vi "Dashboard Main.vi"() -> ()   [LabVIEW 2017]
uses:
  <vilib>/Utility/miscctls.llb/LVRowAndColumnTypeDef.ctl
  <vilib>/Rock Robotics/Network Tables/NT Write Boolean.vi
  <vilib>/Rock Robotics/WPI/Dashboard/WPI_DashboardLogging Global.vi
panel:
  out "timer":sgl(slide) scale=0.0..100.0
  in  "Camera Name":string(combo)="No Camera Selection"
  in  "Camera Settings":T1={"Frame Rate"=30, "Compression"=30, "Size"=1, "DB Camera Config"=FALSE} {"Frame Rate" scale=1.0..30.0; "Compression" scale=100.0..-1.0; "Size" items=["640x480", "320x240", "160x120"]}
  in  "TCP":refnum<k5>
  out "Robot IP":string
  out "Image Message":string="Timeout in Camera Communications"
  in  "Dashboard Tab":T2(tab)
  out "Gyro":dbl(knob) scale=0.0..360.0
  in  "Auto Wait (s)":dbl
  in  "Reverse Climber":bool
  in  "Start Side":i32(listbox)
  in  "Autonomous":i32(listbox)
  out "NT Connection":bool
  out "Mode":T3(ring)=enum."Auto Disabled"
  out "Camera Info":cluster{"Mbps LED":bool, "Mbps":dbl, "fps":dbl} {"fps" format="%#.1g"; "Mbps" format="%#.1g"}
  in  "Rec Mode":enum32{"Stop", "Record", "Playback"}(radio)
  in  "driveRampUpD":dbl
  in  "driveRampUpS":dbl
  in  "driveS3":dbl
  in  "driveD3":dbl
  in  "driveS2":dbl
  in  "turnS2":dbl
  in  "driveD2":dbl
  in  "driveS1":dbl
  in  "turnD2":dbl
  in  "turnS1":dbl
  in  "afterDriveWait":dbl
  in  "outtakeSpeed":dbl
  in  "intakeSpeed":dbl
  in  "climbCurLim":dbl
  in  "rightPos_D":dbl
  in  "rightPos_I":dbl
  in  "rightPos_P":dbl
  in  "leftPos_D":dbl
  in  "leftPos_I":dbl
  in  "leftPos_P":dbl
  in  "turn_D":dbl
  in  "turn_I":dbl
  in  "turn_P":dbl
  in  "rightDrive_F":dbl
  in  "leftDrive_F":dbl
  in  "rightDrive_D":dbl
  in  "rightDrive_I":dbl
  in  "rightDrive_P":dbl
  in  "leftDrive_D":dbl
  in  "leftDrive_I":dbl
  in  "leftDrive_P":dbl
  in  "configFile":path=path "C:/Users/lavre/Desktop/Robotics/Programming/2018 Programming/2018-Dashboard/docs/config_sample.json"
  in  "DB Camera Config":bool
  in  "Camera Settings Right":T4={"Frame Rate"=30, "Compression"=30, "Size"=1} {"Frame Rate" scale=1.0..30.0; "Compression" scale=100.0..-1.0; "Size" items=["640x480", "320x240", "160x120"]}
  in  "Camera Name Right":string(combo)="No Camera Selection"
  in  "Test Slider":dbl(slide) scale=0.0..100.0 scale format="%#_3g"
  in  "On/Off":bool caption="Solenoid"
  in  "Test Name":u16(ring) items=["Select the test to run..."]
  in  "Test Tree":string(tree)
  in  "Motor":cluster{"Value":dbl, "Enable":bool} {"Value" scale=-1.0..1.0 scale format="%#_3g"}
  out "Progress":T5 {"Test Progress" scale=0.0..100.0}
  in  "Rev/Fwd":cluster{"Forward":bool, "Reverse":bool}
  in  "Test Ring":u16(ring) items=["Monochrome", "Color"]
  out "Cmd Status":string
  in  "Execute Command":bool
  in  "Command Params":string[][](table)
  in  "Command Selection":i32(listbox)
  out "Tree":string(tree)
  out "Camera Image":T6(plugin-control)
  # "HW"
  # "Asterisks (*) mean that that auto is untested\nand should not be run in a competition setting"
  # "Velocity PID Constants"
  # "Auto Turn PID Constants"
  # "Auto Drive PID Constants"
  # "Auto Drive Ramp Constants"
  # "Tele-Op Constants"
  # "Auto Turn Ramp Constants"
  # "inches"
  # "Amps"
  # "inches"
  # "inches"
  # "S1: max speed (native units [1-4200])\nS2: bot speed (native units [1-4200])\nD2: angle from target at which to switch to S2 (in)"
  # "ms"
  # "HW"
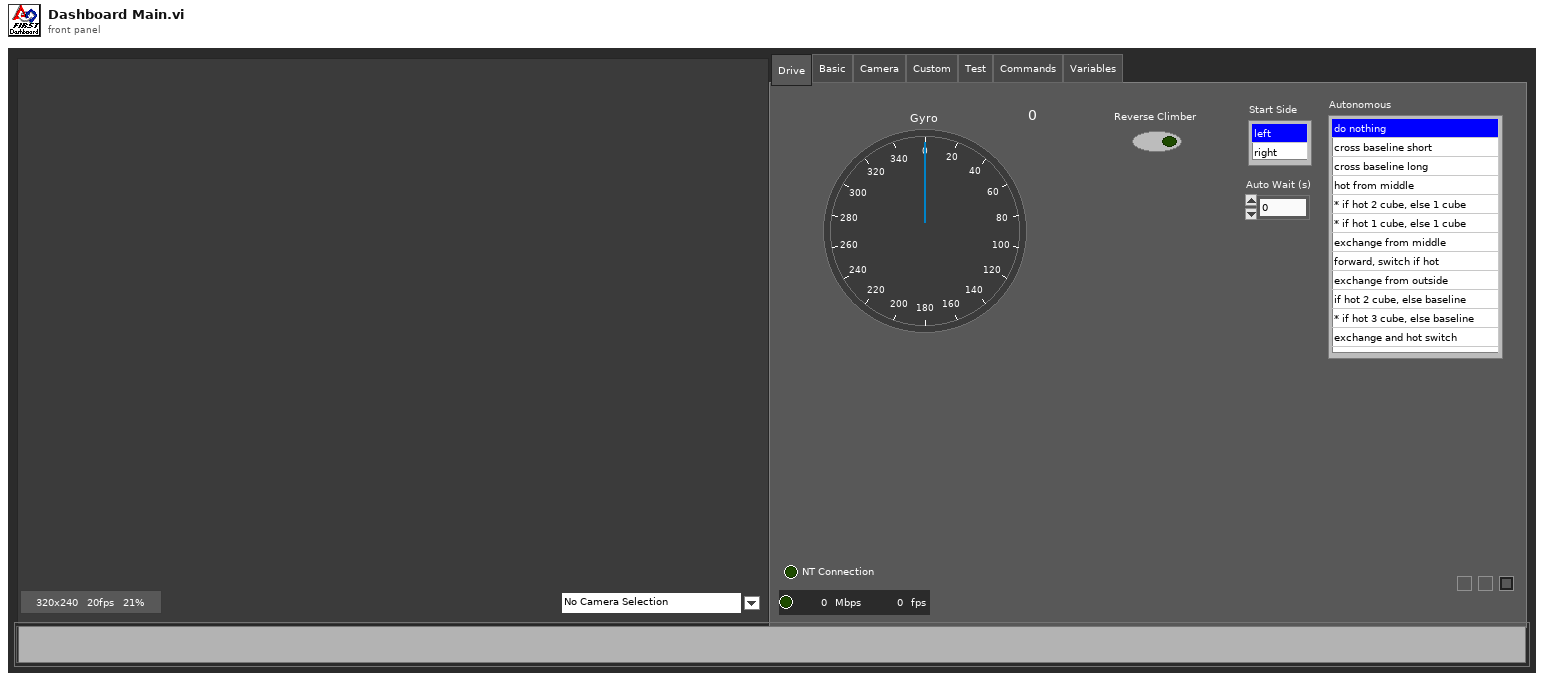
[diagram p1: front panel]
types:
  T1 = cluster{"Frame Rate":i32, "Compression":i32, "Size":u16, "DB Camera Config":bool}
  T2 = enum32{"Drive", "Basic", "Camera", "Custom", "Test", "Commands", "Variables"}
  T3 = enum8{"Tele-Op Disabled", "Tele-Op Enabled", "Auto Disabled", "Auto Enabled", "Test Disabled", "Test Enabled", "Disconnected", "No Code", "E-Stop"}
  T4 = cluster{"Frame Rate":i32, "Compression":i32, "Size":u16}
  T5 = cluster{"Test Progress":u8, "Test Progress Text":string}
  T6 = typedef "IMAQ Image.ctl" = refnum<image>
  T7 = cluster{"Save Path":path, "Interval (s)":dbl, "Keep":i32}
  T8 = enum32{"Drive", "Camera", "Basic", "Custom", "Test", "Commands", "Checklist", "Variables"}
  T9 = typedef "Image Type" = u32
  T10 = cluster{"IDs":cluster{"RPC field ID":u16, "Unique ID":u16}, "String":string}
  T11 = cluster{"velocityPIDConsts":cluster{"leftDrive_P":dbl, "leftDrive_I":dbl, "leftDrive_D":dbl, "leftDrive_F":dbl, "rightDrive_P":dbl, "rightDrive_I":dbl, "rightDrive_D":dbl, "rightDrive_F":dbl}, "teleOpConsts":cluster{"climbCurLim":dbl, "intakeSpeed":dbl, "outtakeSpeed":dbl, "reverseClimber":bool}, "autoTurnPIDConsts":cluster{"turn_P":dbl, "turn_I":dbl, "turn_D":dbl}, "autoTurnRampConsts":cluster{"turnS1":dbl, "turnD2":dbl, "turnS2":dbl}, "autoDrivePIDConsts":cluster{"leftPos_P":dbl, "leftPos_I":dbl, "leftPos_D":dbl, "rightPos_P":dbl, "rightPos_I":dbl, "rightPos_D":dbl}, "autoDriveRampConsts":cluster{"driveS1":dbl, "driveD2":dbl, "driveS2":dbl, "driveD3":dbl, "driveS3":dbl, "autoDriveRampUpS":dbl, "autoDriveRampUpD":dbl, "afterDriveWait":dbl}}
  T12 = cluster{"leftDrive_P":dbl, "leftDrive_I":dbl, "leftDrive_D":dbl, "leftDrive_F":dbl, "rightDrive_P":dbl, "rightDrive_I":dbl, "rightDrive_D":dbl, "rightDrive_F":dbl}
  T13 = cluster{"climbCurLim":dbl, "intakeSpeed":dbl, "outtakeSpeed":dbl, "reverseClimber":bool}
  T14 = cluster{"turn_P":dbl, "turn_I":dbl, "turn_D":dbl}
  T15 = cluster{"turnS1":dbl, "turnD2":dbl, "turnS2":dbl}
  T16 = cluster{"leftPos_P":dbl, "leftPos_I":dbl, "leftPos_D":dbl, "rightPos_P":dbl, "rightPos_I":dbl, "rightPos_D":dbl}
  T17 = cluster{"driveS1":dbl, "driveD2":dbl, "driveS2":dbl, "driveD3":dbl, "driveS3":dbl, "autoDriveRampUpS":dbl, "autoDriveRampUpD":dbl, "afterDriveWait":dbl}
  T18 = cluster{"Error Strings":string, "Disable Counts":cluster{u16, u16}, "Rail Faults":cluster{u16, u16, u16}, "Robot IP":string, "DB Mode":u8, "Event Info":cluster{"Name":string, "Type":u8, "Number":u16, "Replay":u8}}
  T19 = cluster{"Storage":cluster{"Disk Free":u64, "RAM Block":u32, "RAM free":u32}, "CPU Utilization":cluster{"CPU % ISR":sgl, "CPU % Time Crit":sgl, "CPU % Timed Str":sgl, "CPU % High":sgl, "CPU % Above":sgl, "CPU % Normal":sgl, "CPU % Low":sgl}, "CAN":cluster{"% Bus Utilization":sgl, "Bus Off Cnt":u32, "TX_FIFO Full Cnt":u32, "Receive Error Cnt":u8, "Transmit Error Cnt":u8}, "HID":cluster{"HID Outputs":u32, "Rumble Low":u16, "Rumble High":u16}[]}
  T20 = cluster{"Status bits":cluster{"Test Mode":bool, "Autonomous":bool, "Enabled":bool, "Code Start":bool, "Brownout":bool, "Reserved 2":bool, "Reserved 3":bool, "E-Stop":bool}, "Code Trace":cluster{"Disabled":bool, "TeleOp":bool, "Auto":bool, "Test":bool}, "Controller Type":enum16{"unknown", "cRIO", "roboRio"}, "Code?":enum16{"unknown", "noCode", "code"}, "Battery V":dbl}
  T21 = cluster{"Control Bits":cluster{"TestMode":bool, "Autonomous":bool, "Enabled":bool, "FMS Present":bool, bool, bool, bool, "E-Stop":bool}, "Team Station ":u8, "Countdown":sgl, "Joystick Values":cluster{"Axes":dbl[], "Buttons":bool[], "POVs":i16[]}[]}
  T22 = cluster{"Camera Name":string, string, "Saved DB Images Info":cluster{"Save Path":path, "Interval (s)":dbl, "Keep":i32}}
  T23 = cluster{"Camera Name Right":string, string, "Saved DB Images Info":cluster{"Save Path":path, "Interval (s)":dbl, "Keep":i32}}
  T24 = cluster{"Operation":enum16{"Update", "Clear"}, "Color Box":u32}[]
  T25 = cluster{"Image Size":bool, "Image Type":bool, "Pixel Value":bool, "ROI Information":bool, "Zoom Factor":bool}
  T26 = cluster{"Operation":enum16{"Update", "Clear"}, "Color Box":u32}
  T27 = typedef "LVRowAndColumnTypeDef.ctl" = cluster{"Row":i32, "Column":i32}
  T28 = cluster{"Shift":bool, "Ctrl":bool, "Alt":bool, "Cmd":bool, "Opt":bool}
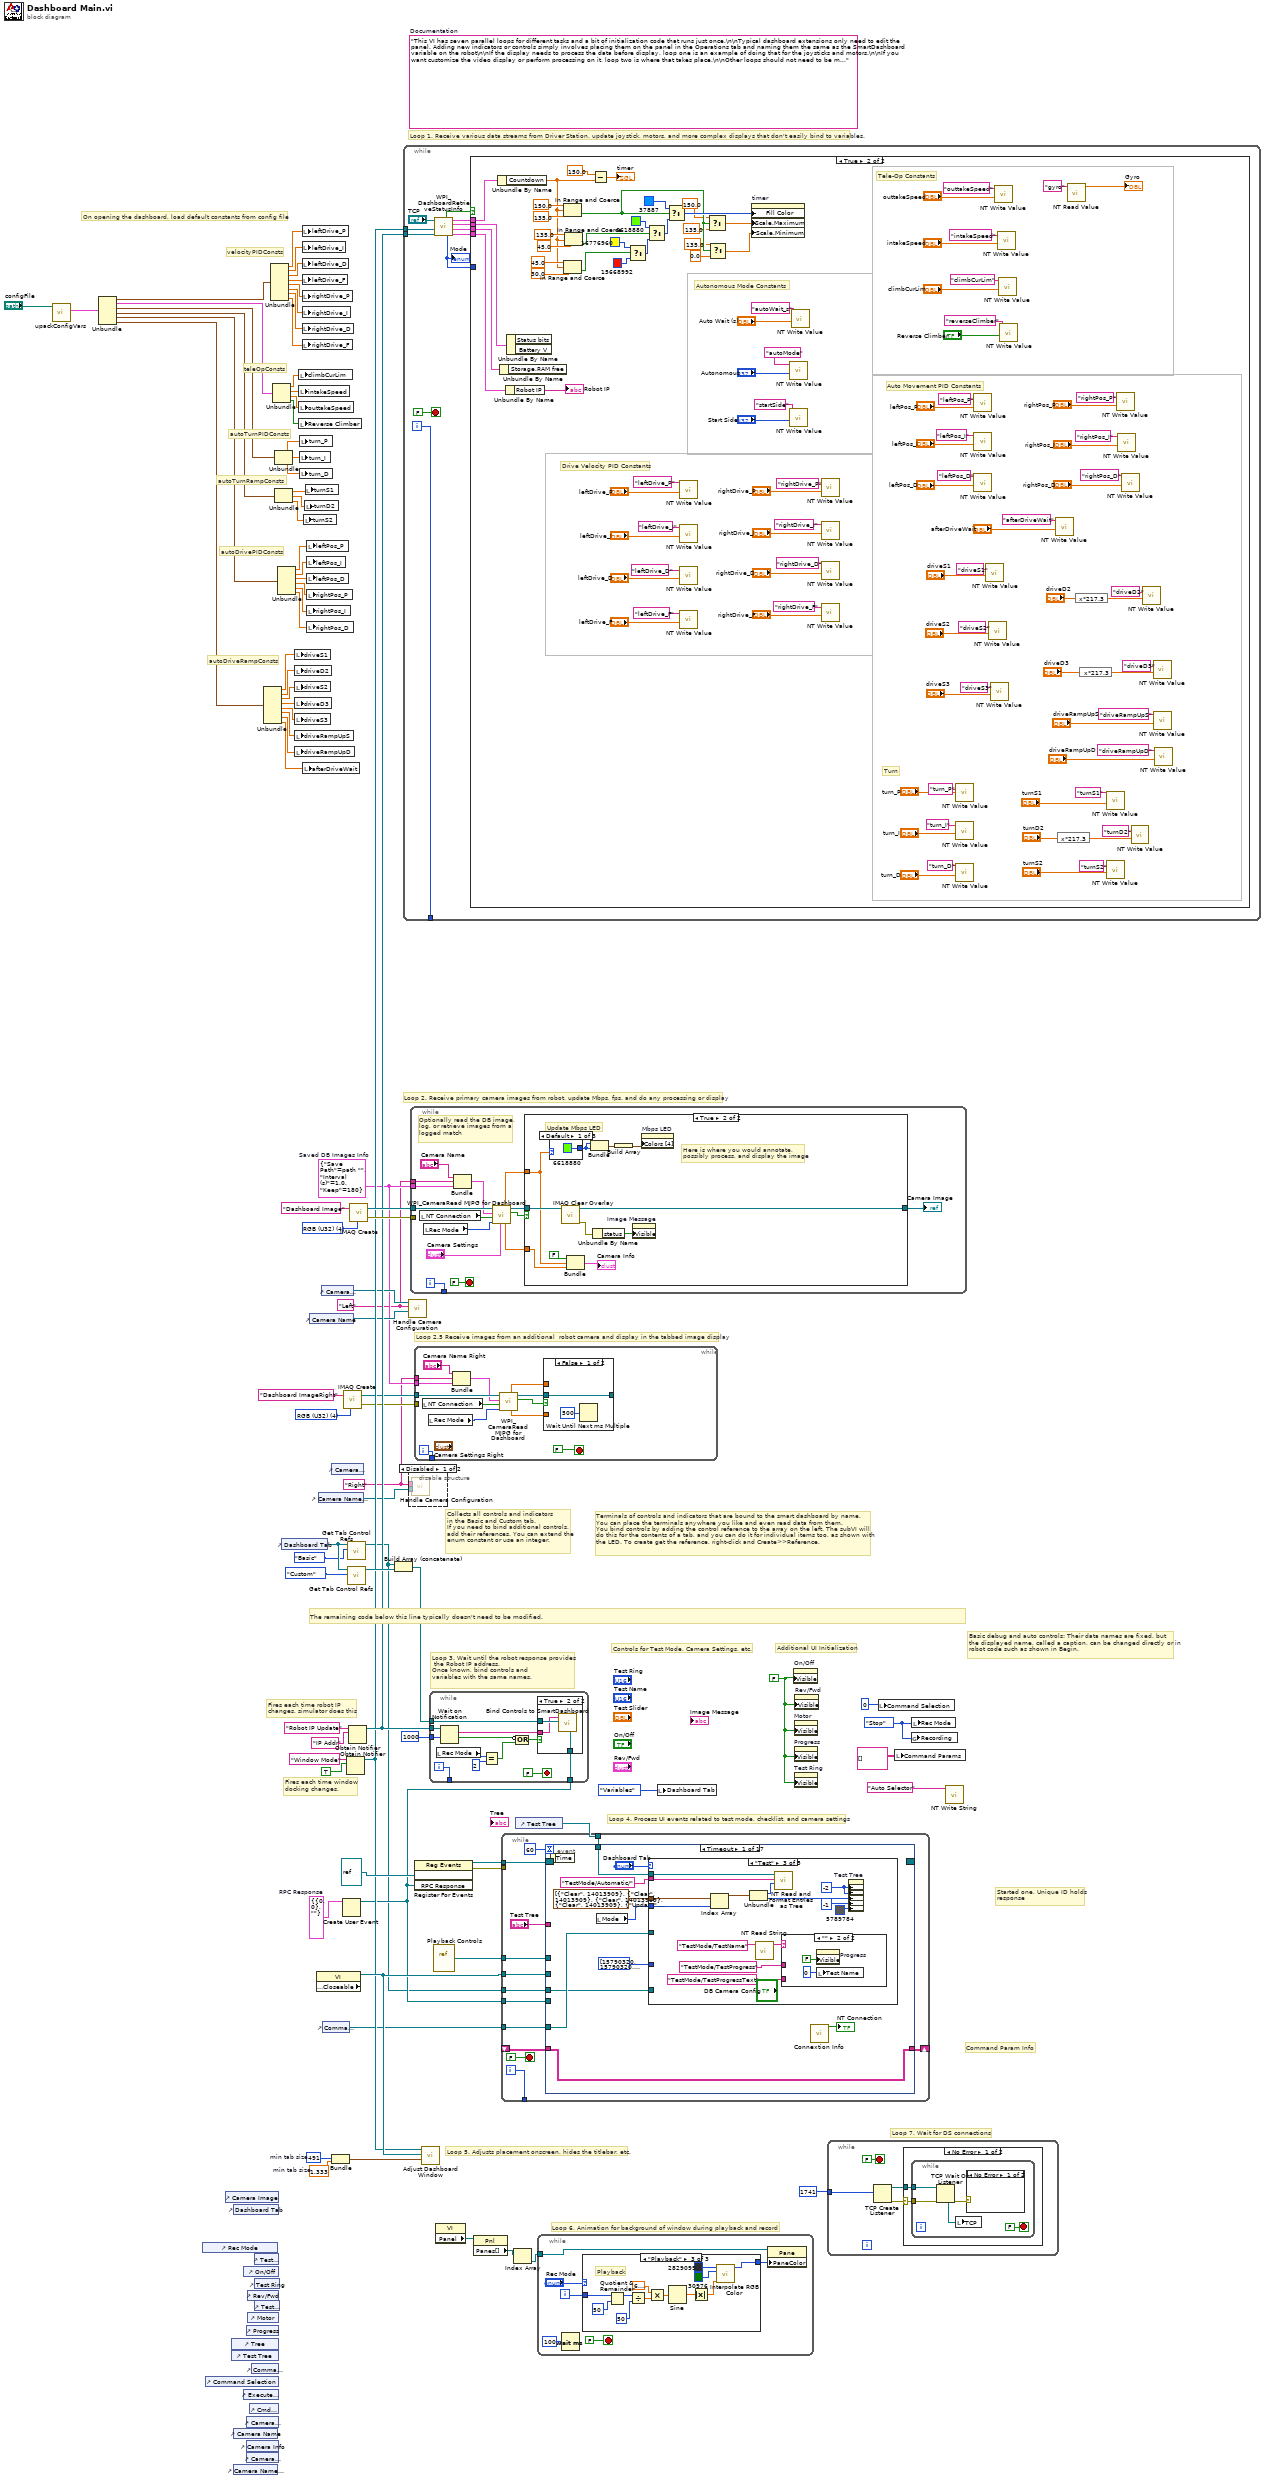
[diagram p0: block diagram]
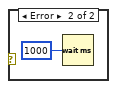
[diagram p4: hidden frame]
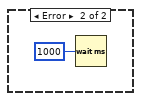
[diagram p5: hidden frame]
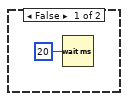
[diagram p6: hidden frame]
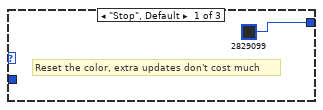
[diagram p7: hidden frame]
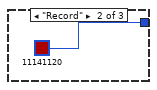
[diagram p8: hidden frame]
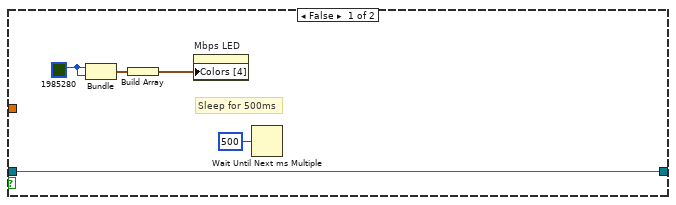
[diagram p10: hidden frame]
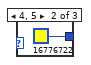
[diagram p11: hidden frame]
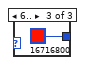
[diagram p12: hidden frame]
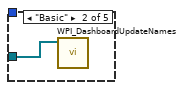
[diagram p14: hidden frame]
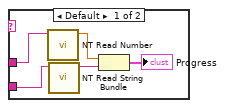
[diagram p15: hidden frame]
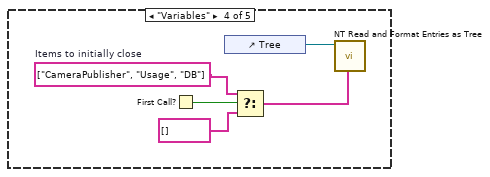
[diagram p16: hidden frame]
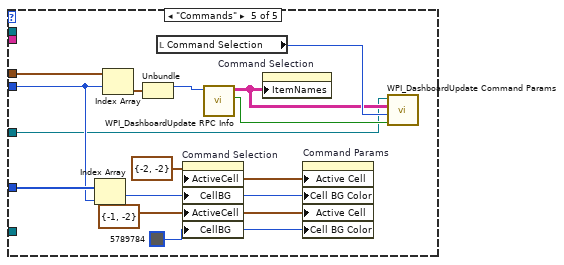
[diagram p17: hidden frame]
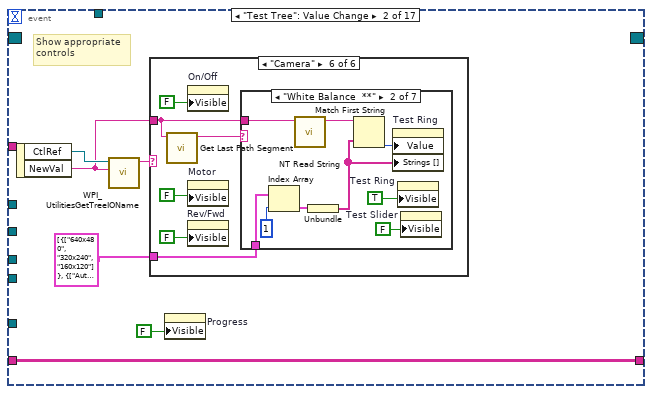
[diagram p18: hidden frame]
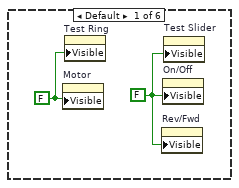
[diagram p19: hidden frame]
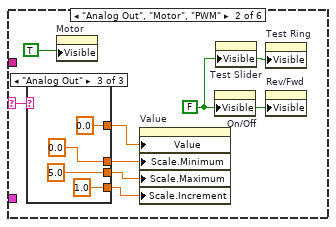
[diagram p20: hidden frame]
diagram:
  w43 = T7 {"Save Path"=path "", "Interval (s)"=1.0, "Keep"=180}  # Saved DB Images Info
  w42 = "Right"
  w41 = "Left"
  w49 = T9 4 items=["Grayscale (U8)", "Grayscale (I16)", "Grayscale (SGL)", "Complex (CSG)", "RGB (U32)", "HSL (U32)", "RGB (U64)"] ("Image Type")
  w59 = T10 {"IDs"={"RPC field ID"=0, "Unique ID"=0}, "String"=""}  # RPC Response
  w67 = 491  # min tab size
  w66 = 1.333  # min tab size
  w72 = enum32{"Stop", "Record", "Playback"}."Stop" ("Rec Mode")
  w64 = FALSE ("Visible")
  (unwired) "This VI has seven parallel loops for different tasks and a bit of initialization code that runs just once.\n\nTypical dashboard extensions only need to edit the panel. Adding new indicators or controls simply involves placing them on the panel in the Operations tab and naming them the same as the SmartDashboard variable on the robot\n\nIf the display needs to process the data before display, loop one is an example of doing that for the joysticks and motors.\n\nIf you want customize the video display or perform processing on it, loop two is where that takes place.\n\nOther loops should not need to be modified. They are pretty standard, and document the task they perform."  # Documentation
  w89 = T9 4 items=["Grayscale (U8)", "Grayscale (I16)", "Grayscale (SGL)", "Complex (CSG)", "RGB (U32)", "HSL (U32)", "RGB (U64)"] ("Image Type")
  # "autoDriveRampConsts"
  # "autoDrivePIDConsts"
  # "autoTurnRampConsts"
  # "autoTurnPIDConsts"
  # "teleOpConsts"
  # "velocityPIDConsts"
  # "On opening the dashboard, load default constants from config file"
  # "Collects all controls and indicators\nin the Basic and Custom tab.\nIf you need to bind additional controls,\nadd their references. You can extend the\nenum constant or use an integer."
  # "Loop 2.5 Receive images from an additional  robot camera and display in the tabbed image display"
  # "Command Param Info"
  # "Started one, Unique ID holds\nresponse"
  # "Loop 7. Wait for DS connections"
  # "Basic debug and auto controls: Their data names are fixed, but\nthe displayed name, called a caption, can be changed directly or in\nrobot code such as shown in Begin."
  # "Controls for Test Mode, Camera Settings, etc."
  # "Additional UI Initialization"
  # "Loop 6. Animation for background of window during playback and record"
  # "Fires each time robot IP\nchanges, simulator does this"
  # "Fires each time window\ndocking changes."
  # "The remaining code below this line typically doesn't need to be modified."
  # "Loop 4. Process UI events related to test mode, checklist, and camera settings"
  # "Terminals of controls and indicators that are bound to the smart dashboard by name.\nYou can place the terminals anywhere you like and even read data from them.\nYou bind controls by adding the control reference to the array on the left. The subVI will\ndo this for the contents of a tab, and you can do it for individual items too, as shown with\nthe LED. To create get the reference, right-click and Create>>Reference."
  # "Loop 3. Wait until the robot response provides\n the Robot IP address.\nOnce known, bind controls and\nvariables with the same names."
  # "Loop 5. Adjusts placement onscreen, hides the titlebar, etc."
  # "Loop 1. Receive various data streams from Driver Station, update joystick, motors, and more complex displays that don't easily bind to variables."
  # "Loop 2. Receive primary camera images from robot, update Mbps, fps, and do any processing or display"
  n1 = call "upackConfigVars.vi"("file"="configFile") -> ("configVars"=w1:T11)  [unwired: 10 in]
  n2 = Unbundle(w1) -> ("velocityPIDConsts"=w31:T12, "teleOpConsts"=w30:T13, "autoTurnPIDConsts"=w25:T14, "autoTurnRampConsts"=w21:T15, "autoDrivePIDConsts"=w17:T16, "autoDriveRampConsts"=w16:T17)
  n3 = control-ref of="Rec Mode"() -> ()  [unwired: 1 out]
  n4 = control-ref of="Command Selection"() -> ()  [unwired: 1 out]
  n5 = control-ref of="Camera Image"() -> ()  [unwired: 1 out]
  n6 = control-ref of="Tree"() -> ()  [unwired: 1 out]
  n7 = control-ref of="Test Tree"() -> ()  [unwired: 1 out]
  n8 = control-ref of="Dashboard Tab"() -> ()  [unwired: 1 out]
  n9 = control-ref of="Camera Name"() -> ()  [unwired: 1 out]
  n10 = control-ref of="Camera Name Right"() -> ()  [unwired: 1 out]
  n11 = control-ref of="Execute Command"() -> ()  [unwired: 1 out]
  n12 = control-ref of="On/Off"() -> ()  [unwired: 1 out]
  n13 = control-ref of="Progress"() -> ()  [unwired: 1 out]
  n14 = control-ref of="Camera Settings"() -> ()  [unwired: 1 out]
  n15 = control-ref of="Camera Info"() -> ()  [unwired: 1 out]
  n16 = control-ref of="Camera Settings Right"() -> ()  [unwired: 1 out]
  n17 = control-ref of="Rev/Fwd"() -> ()  [unwired: 1 out]
  n18 = control-ref of="Motor"() -> ()  [unwired: 1 out]
  n19 = control-ref of="Cmd Status"() -> ()  [unwired: 1 out]
  n20 = control-ref of="Command Params"() -> ()  [unwired: 1 out]
  n21 = control-ref of="Test Slider"() -> ()  [unwired: 1 out]
  n22 = control-ref of="Test Ring"() -> ()  [unwired: 1 out]
  n23 = control-ref of="Test Name"() -> ()  [unwired: 1 out]
  n24 = Unbundle(w16) -> ("driveS1"=w2:dbl, "driveD2"=w3:dbl, "driveS2"=w4:dbl, "driveD3"=w5:dbl, "driveS3"=w6:dbl, "autoDriveRampUpS"=w7:dbl, "autoDriveRampUpD"=w8:dbl, "afterDriveWait"=w9:dbl)
  n25 = Unbundle(w31) -> ("leftDrive_P"=w39:dbl, "leftDrive_I"=w38:dbl, "leftDrive_D"=w37:dbl, "leftDrive_F"=w36:dbl, "rightDrive_P"=w35:dbl, "rightDrive_I"=w34:dbl, "rightDrive_D"=w33:dbl, "rightDrive_F"=w32:dbl)
  n26 = Unbundle(w30) -> ("climbCurLim"=w29:dbl, "intakeSpeed"=w28:dbl, "outtakeSpeed"=w27:dbl, "reverseClimber"=w26:bool)
  n27 = Unbundle(w25) -> ("turn_P"=w24:dbl, "turn_I"=w23:dbl, "turn_D"=w22:dbl)
  n28 = Unbundle(w21) -> ("turnS1"=w20:dbl, "turnD2"=w18:dbl, "turnS2"=w19:dbl)
  n29 = Unbundle(w17) -> ("leftPos_P"=w15:dbl, "leftPos_I"=w14:dbl, "leftPos_D"=w12:dbl, "rightPos_P"=w13:dbl, "rightPos_I"=w11:dbl, "rightPos_D"=w10:dbl)
  n30 = control-ref of="Dashboard Tab"() -> (w70:refnum<vi>)
  n31 = local write "driveS1"(w2) -> ()
  n32 = local write "driveD2"(w3) -> ()
  n33 = local write "driveS2"(w4) -> ()
  n34 = local write "driveD3"(w5) -> ()
  n35 = local write "driveS3"(w6) -> ()
  n36 = local write "driveRampUpS"(w7) -> ()
  n37 = local write "driveRampUpD"(w8) -> ()
  n38 = local write "climbCurLim"(w29) -> ()
  n39 = local write "intakeSpeed"(w28) -> ()
  n40 = local write "outtakeSpeed"(w27) -> ()
  n41 = local write "Reverse Climber"(w26) -> ()
  n42 = local write "turn_P"(w24) -> ()
  n43 = local write "turn_I"(w23) -> ()
  n44 = local write "turn_D"(w22) -> ()
  n45 = local write "leftDrive_P"(w39) -> ()
  n46 = local write "leftDrive_I"(w38) -> ()
  n47 = local write "leftDrive_D"(w37) -> ()
  n48 = local write "leftDrive_F"(w36) -> ()
  n49 = local write "rightDrive_P"(w35) -> ()
  n50 = local write "rightDrive_I"(w34) -> ()
  n51 = local write "rightDrive_D"(w33) -> ()
  n52 = local write "rightDrive_F"(w32) -> ()
  n53 = local write "afterDriveWait"(w9) -> ()
  n54 = local write "turnS2"(w19) -> ()
  n55 = local write "turnD2"(w18) -> ()
  n56 = local write "turnS1"(w20) -> ()
  n57 = local write "leftPos_P"(w15) -> ()
  n58 = local write "leftPos_I"(w14) -> ()
  n59 = local write "leftPos_D"(w12) -> ()
  n60 = local write "rightPos_P"(w13) -> ()
  n61 = local write "rightPos_I"(w11) -> ()
  n62 = local write "rightPos_D"(w10) -> ()
  n63 = control-ref of="Camera Name"() -> (w53:refnum<vi>)
  n64 = property class="VI" props=["Front Panel.Closeable"]() -> (reference out=w71:refnum<vi>)  [unwired: 2 in, 2 out]
  n65 = control-ref of="Camera Name Right"() -> (w46:refnum<vi>)
  n66 = control-ref of="Camera Settings"() -> (w54:refnum<vi>)
  n67 = control-ref of="Command Params"() -> (w55:refnum<vi>)
  n68 = control-ref of="Camera Settings Right"() -> ()  [unwired: 1 out]
  n69 = Bundle("min tab size"=w67, "min tab size"=w66) -> (w65:cluster{"min tab size":i32, "min tab size":dbl})  [unwired: 1 in]
  n70 = Create User Event(user event datatype=w59) -> (user event=w56:refnum<user-event>)  [unwired: 1 in, 1 out]
  n71 = call "IMAQ Create"("Image Name"="Dashboard ImageRight", "Image Type"=w49) -> ("New Image"=w48:T6, "error out"=w47:errorcluster)  [unwired: 2 in, 1 out]
  n72 = Obtain Notifier(name (unnamed)="Window Mode", notification data type=TRUE) -> (notifier out=w62:refnum<notifier>)  [unwired: 2 in, 2 out]
  n73 = call <vilib>:"Get Tab Control Refs.vi"("Page Index"=T8."Basic" ("Dashboard Tab"), "TabControl in"=w70) -> ("ControlsOnPage"=w52:refnum<vi>[])  [unwired: 9 in]
  n74 = call <vilib>:"Get Tab Control Refs.vi"("Page Index"=T8."Custom" ("Dashboard Tab"), "TabControl in"=w70) -> ("ControlsOnPage"=w69:refnum<vi>[])  [unwired: 9 in]
  n75 = Obtain Notifier(name (unnamed)="Robot IP Update", notification data type="IP Addr" ("name (unnamed)")) -> (notifier out=w63:refnum<notifier>)  [unwired: 2 in, 2 out]
  n76 = call "IMAQ Create"("Image Name"="Dashboard Image", "Image Type"=w89) -> ("New Image"=w87:T6, "error out"=w86:errorcluster)  [unwired: 2 in, 1 out]
  n77 = Build Array (concatenate)(w52, w69) -> (w68:refnum<vi>[])
  n78 = while {
    tunnel: [w99] -> _
    tunnel: w63 -> [w93]
    tunnel: w62 -> [w90]
    i -> [w99]
    stop <- FALSE stop-if-true
    n79 = call <vilib>:"WPI_DashboardRetrieveStatusInfo.vi"("Binding Refnum"=w93, "Window Mode Notifier"=w90, "TCP Cnx"="TCP") -> ("Power and Errors"=w94:T18, "Robot Metrics"=w97:T19, "Status Info"=w98:T20, "Control Info"=w95:T21, "Robot Mode"=w92:T3, "Process?"=w96:bool)  [unwired: 3 in]
    "Mode" <- w92
    n80 = case shown="True" w96 {
      tunnel: w98 -> [_ w206]
      tunnel: w97 -> [_ w205]
      tunnel: w95 -> [_ w204]
      tunnel: w94 -> [_ w203]
      tunnel: w92 -> [_ _]
      frame False {
        n81 = Wait (ms)(milliseconds to wait=u32 20) -> ()  [unwired: 1 out]
      }
      frame True {
        # "Turn"
        # "Auto Movement PID Constants"
        # "Drive Velocity PID Constants"
        # "Autonomous Mode Constants"
        # "Tele-Op Constants"
        n82 = Unbundle By Name(w204) -> ("Countdown"=w178:sgl)
        n83 = Unbundle By Name(w205) -> ()  [unwired: 1 out]
        n84 = Unbundle By Name(w203) -> ("Robot IP"=→"Robot IP":string)
        n85 = Unbundle By Name(w206) -> ()  [unwired: 2 out]
        n86 = In Range and Coerce(upper limit=150.0, x=w178, lower limit=135.0) -> (In Range?=w184:bool)  [unwired: 1 out]
        n87 = In Range and Coerce(upper limit=45.0, x=w178, lower limit=30.0) -> (In Range?=w189:bool)  [unwired: 1 out]
        n88 = In Range and Coerce(upper limit=135.0, x=w178, lower limit=45.0) -> (In Range?=w188:bool)  [unwired: 1 out]
        n89 = Subtract(x=sgl 150.0, y=w178) -> (x-y=→"timer":sgl)
        n90 = Select(t=u32 16776960 ("Color Box"), s=w189, f=u32 15668992 ("Color Box")) -> (s? t:f=w196:u32)
        n91 = Select(t=u32 6618880 ("Color Box"), s=w188, f=w196) -> (s? t:f=w198:u32)
        n92 = Select(t=u32 37887 ("Color Box"), s=w184, f=w198) -> (s? t:f=w187:u32)
        n93 = call-poly <vilib>:"NT Write Value.vi"("Numeric"="leftDrive_P", "Name"="leftDrive_P") -> ()  [unwired: 9 in, 1 out]
        n94 = call-poly <vilib>:"NT Write Value.vi"("Numeric"="leftDrive_I", "Name"="leftDrive_I") -> ()  [unwired: 9 in, 1 out]
        n95 = call-poly <vilib>:"NT Write Value.vi"("Numeric"="leftDrive_D", "Name"="leftDrive_D") -> ()  [unwired: 9 in, 1 out]
        n96 = call-poly <vilib>:"NT Write Value.vi"("Numeric"="leftDrive_F", "Name"="leftDrive_F") -> ()  [unwired: 9 in, 1 out]
        n97 = Select(t=150.0, s=w184, f=135.0) -> (s? t:f=w186:dbl)
        n98 = Select(t=135.0, s=w184, f=0.0) -> (s? t:f=w185:dbl)
        n99 = property on="timer" class="Slide (strict)"("Fill Color"=w187, "Scale.Maximum"=w186, "Scale.Minimum"=w185) -> ()  [unwired: 2 in, 2 out]
        n100 = call-poly <vilib>:"NT Write Value.vi"("Numeric"="Autonomous", "Name"="autoMode") -> ()  [unwired: 9 in, 1 out]
        n101 = call-poly <vilib>:"NT Write Value.vi"("Numeric"="Start Side", "Name"="startSide") -> ()  [unwired: 9 in, 1 out]
        n102 = call-poly <vilib>:"NT Write Value.vi"("Numeric"="Auto Wait (s)", "Name"="autoWait_s") -> ()  [unwired: 9 in, 1 out]
        n103 = call-poly <vilib>:"NT Write Value.vi"("Numeric"="rightDrive_P", "Name"="rightDrive_P") -> ()  [unwired: 9 in, 1 out]
        n104 = call-poly <vilib>:"NT Write Value.vi"("Numeric"="rightDrive_I", "Name"="rightDrive_I") -> ()  [unwired: 9 in, 1 out]
        n105 = call-poly <vilib>:"NT Write Value.vi"("Numeric"="rightDrive_D", "Name"="rightDrive_D") -> ()  [unwired: 9 in, 1 out]
        n106 = call-poly <vilib>:"NT Write Value.vi"("Numeric"="rightDrive_F", "Name"="rightDrive_F") -> ()  [unwired: 9 in, 1 out]
        n107 = call-poly <vilib>:"NT Write Value.vi"("Numeric"="turn_P", "Name"="turn_P") -> ()  [unwired: 9 in, 1 out]
        n108 = call-poly <vilib>:"NT Write Value.vi"("Numeric"="turn_I", "Name"="turn_I") -> ()  [unwired: 9 in, 1 out]
        n109 = call-poly <vilib>:"NT Write Value.vi"("Numeric"="turn_D", "Name"="turn_D") -> ()  [unwired: 9 in, 1 out]
        n110 = call-poly <vilib>:"NT Write Value.vi"("Numeric"="leftPos_P", "Name"="leftPos_P") -> ()  [unwired: 9 in, 1 out]
        n111 = call-poly <vilib>:"NT Write Value.vi"("Numeric"="leftPos_I", "Name"="leftPos_I") -> ()  [unwired: 9 in, 1 out]
        n112 = call-poly <vilib>:"NT Write Value.vi"("Numeric"="leftPos_D", "Name"="leftPos_D") -> ()  [unwired: 9 in, 1 out]
        n113 = call-poly <vilib>:"NT Write Value.vi"("Numeric"="driveS1", "Name"="driveS1") -> ()  [unwired: 9 in, 1 out]
        n114 = call-poly <vilib>:"NT Write Value.vi"("Numeric"="driveS2", "Name"="driveS2") -> ()  [unwired: 9 in, 1 out]
        n115 = call-poly <vilib>:"NT Write Value.vi"("Numeric"="driveS3", "Name"="driveS3") -> ()  [unwired: 9 in, 1 out]
        n116 = call-poly <vilib>:"NT Write Value.vi"("Numeric"="outtakeSpeed", "Name"="outtakeSpeed") -> ()  [unwired: 9 in, 1 out]
        n117 = call-poly <vilib>:"NT Write Value.vi"("Numeric"="intakeSpeed", "Name"="intakeSpeed") -> ()  [unwired: 9 in, 1 out]
        n118 = call-poly <vilib>:"NT Write Value.vi"("Numeric"="climbCurLim", "Name"="climbCurLim") -> ()  [unwired: 9 in, 1 out]
        n119 = call-poly <vilib>:"NT Write Value.vi"("Boolean"="Reverse Climber", "Name"="reverseClimber") -> ()  [unwired: 9 in, 1 out]
        n120 = call-poly <vilib>:"NT Write Value.vi"("Numeric"="afterDriveWait", "Name"="afterDriveWait") -> ()  [unwired: 9 in, 1 out]
        n121 = expression code="x*217.3"("turnD2") -> (w102:dbl)
        n122 = call-poly <vilib>:"NT Read Value.vi"("Name"="gyro") -> ("Numeric"=→"Gyro":dbl)  [unwired: 9 in, 1 out]
        n123 = expression code="x*217.3"("driveD2") -> (w106:dbl)
        n124 = expression code="x*217.3"("driveD3") -> (w104:dbl)
        n125 = call-poly <vilib>:"NT Write Value.vi"("Numeric"="turnS1", "Name"="turnS1") -> ()  [unwired: 9 in, 1 out]
        n126 = call-poly <vilib>:"NT Write Value.vi"("Numeric"="turnS2", "Name"="turnS2") -> ()  [unwired: 9 in, 1 out]
        n127 = call-poly <vilib>:"NT Write Value.vi"("Numeric"="rightPos_P", "Name"="rightPos_P") -> ()  [unwired: 9 in, 1 out]
        n128 = call-poly <vilib>:"NT Write Value.vi"("Numeric"="rightPos_I", "Name"="rightPos_I") -> ()  [unwired: 9 in, 1 out]
        n129 = call-poly <vilib>:"NT Write Value.vi"("Numeric"="rightPos_D", "Name"="rightPos_D") -> ()  [unwired: 9 in, 1 out]
        n130 = call-poly <vilib>:"NT Write Value.vi"("Numeric"=w102, "Name"="turnD2") -> ()  [unwired: 9 in, 1 out]
        n131 = call-poly <vilib>:"NT Write Value.vi"("Numeric"=w106, "Name"="driveD2") -> ()  [unwired: 9 in, 1 out]
        n132 = call-poly <vilib>:"NT Write Value.vi"("Numeric"=w104, "Name"="driveD3") -> ()  [unwired: 9 in, 1 out]
        n133 = call-poly <vilib>:"NT Write Value.vi"("Numeric"="driveRampUpS", "Name"="driveRampUpS") -> ()  [unwired: 9 in, 1 out]
        n134 = call-poly <vilib>:"NT Write Value.vi"("Numeric"="driveRampUpD", "Name"="driveRampUpD") -> ()  [unwired: 9 in, 1 out]
      }
    }
  }
  n135 = call "Handle Camera Configuration.vi"("CameraNameRef"=w53, "Display Name"=w41, "ClusterRef"=w54) -> ()  [unwired: 9 in]
  n136 = disable-structure shown="Disabled" {
    disable-tunnel: w46 -> [w208 _]
    disable-tunnel: w42 -> [w207 _]
    frame Disabled {
      n137 = call "Handle Camera Configuration.vi"("CameraNameRef"=w208, "Display Name"=w207) -> ()  [unwired: 10 in]
    }
    frame Enabled {
    }
  }
  n138 = while {
    tunnel: w87 -> [w221]
    tunnel: w86 -> [_]
    tunnel: [w222] -> _
    tunnel: w43 -> [w212]
    tunnel: w41 -> [w209]
    i -> [w222]
    stop <- FALSE stop-if-true
    # "Optionally read the DB image,\nlog, or retrieve images from a\nlogged match"
    n139 = local read "NT Connection"() -> (w213:bool)
    n140 = local read "Rec Mode"() -> (w217:enum32{"Stop", "Record", "Playback"})
    n141 = Bundle("Camera Name"="Camera Name", w209, "Saved DB Images Info"=w212) -> (w211:T22)  [unwired: 1 in]
    n142 = call <vilib>:"WPI_CameraRead MJPG for Dashboard.vi"("Camera Settings"="Camera Settings", "Rec Mode"=w217, "NT Connection"=w213, "Capture Info"=w211, "Refnum in"=w221) -> ("Active"=w219:bool, "Refnum out"=w220:T6, "FPS"=w218:dbl, "Bandwidth (Mbps)"=w216:dbl)  [unwired: 3 in]
    n143 = case shown="True" w219 {
      tunnel: w220 -> [w224 w235]
      tunnel: w216 -> [_ w232]
      tunnel: w218 -> [_ w233]
      tunnel: [w224 w229] -> w214
      frame False {
        w226 = u32 1985280 ("Color Box")
        # "Sleep for 500ms"
        n144 = Bundle("Color Box"=w226, "Color Box"=w226) -> (w227:cluster{"Color Box":u32, "Color Box":u32})  [unwired: 1 out]
        n145 = Build Array(w227) -> (w225:cluster{"Color Box":u32, "Color Box":u32}[])
        n146 = property on="Mbps LED" class="Bool (strict)"("Colors [4]"=w225) -> ()  [unwired: 2 in, 2 out]
        n147 = Wait Until Next ms Multiple(millisecond multiple=u32 500) -> ()  [unwired: 1 out]
      }
      frame True {
        # "Here is where you would annotate,\npossibly process, and display the image"
        # "Update Mbps LED"
        n148 = case shown="Default" w232 {
          tunnel: [u32 6618880 ("Color Box") u32 16776722 ("Color Box") u32 16716800 ("Color Box")] -> w236
          frame Default {
          }
          frame 4, 5 {
          }
          frame 6.. {
          }
        }
        n149 = call "IMAQ Clear Overlay"("Image"=w235) -> ("error out"=w238:errorcluster, "Image Out"=w229:T6)  [unwired: 2 in, 7 out]
        n150 = Bundle(FALSE, "Bandwidth (Mbps)"=w232, "FPS"=w233) -> (→"Camera Info":cluster{bool, "Bandwidth (Mbps)":dbl, "FPS":dbl})  [unwired: 1 in]
        n151 = Bundle("Color Box"=w236, "Color Box"=w236) -> (w237:cluster{"Color Box":u32, "Color Box":u32})  [unwired: 1 out]
        n152 = Unbundle By Name(w238) -> ("status"=w239:bool)
        n153 = Build Array(w237) -> (w234:cluster{"Color Box":u32, "Color Box":u32}[])
        n154 = property on="Image Message" class="Str"("Visible"=w239) -> ()  [unwired: 2 in, 2 out]
        n155 = property on="Mbps LED" class="Bool (strict)"("Colors [4]"=w234) -> ()  [unwired: 2 in, 2 out]
      }
    }
    "Camera Image" <- w214
  }
  n156 = while {
    tunnel: w48 -> [w255]
    tunnel: w47 -> [_]
    tunnel: [w251] -> _
    tunnel: w43 -> [w246]
    tunnel: w42 -> [w243]
    i -> [w251]
    stop <- FALSE stop-if-true
    n157 = local read "NT Connection"() -> (w247:bool)
    n158 = local read "Rec Mode"() -> (w254:enum32{"Stop", "Record", "Playback"})
    n159 = Bundle("Camera Name Right"="Camera Name Right", w243, "Saved DB Images Info"=w246) -> (w245:T23)  [unwired: 1 in]
    n160 = call <vilib>:"WPI_CameraRead MJPG for Dashboard.vi"("Rec Mode"=w254, "NT Connection"=w247, "Capture Info"=w245, "Refnum in"=w255) -> ("Active"=w250:bool, "Refnum out"=w253:T6, "FPS"=w248:dbl, "Bandwidth (Mbps)"=w249:dbl)  [unwired: 4 in]
    n161 = case shown="False" w250 {
      tunnel: w253 -> [w256 w258]
      tunnel: w249 -> [_ _]
      tunnel: w248 -> [_ _]
      tunnel: [w256 w258] -> _
      frame False {
        n162 = Wait Until Next ms Multiple(millisecond multiple=u32 500) -> ()  [unwired: 1 out]
      }
      frame True {
      }
    }
  }
  n163 = register-events(refnum<vi> refnum, w56) -> (reference out=w76:refnum<event-registration>, error out=w75:errorcluster)  [unwired: 2 in]
  n164 = call "Adjust Dashboard Window.vi"("Size Constraints"=w65, "VI"=w71, "WIn Mode"=w62) -> ()  [unwired: 9 in]
  n165 = while {
    tunnel: w68 -> [w270]
    tunnel: w63 -> [w268]
    tunnel: [w266] -> _
    tunnel: u32 1000 ("milliseconds to wait") -> [w265]
    tunnel: w56 -> [w259]
    i -> [w266]
    stop <- FALSE stop-if-true
    n166 = local read "Rec Mode"() -> (w261:enum32{"Stop", "Record", "Playback"})
    n167 = Wait on Notification(notifier=w268, timeout in ms (-1)=w265) -> (notification=w267:string, timed out?=w263:bool)  [unwired: 2 in, 2 out]
    n168 = Equal?(x=w261, y=u16 2 ("Rec Mode")) -> (x = y?=w262:bool)
    n169 = Compound Arithmetic op=OR(invert w263, w262) -> (w264:bool)
    n170 = case shown="True" w264 {
      tunnel: w270 -> [_ w273]
      tunnel: w267 -> [_ w272]
      tunnel: w259 -> [_ w271]
      frame False {
      }
      frame True {
        n171 = call <vilib>:"Bind Controls to SmartDashboard.vi"("RPC ref"=w271, "Bound Control Refs"=w273, "Server IP Address"=w272) -> ()  [unwired: 9 in]
      }
    }
  }
  n172 = vi-ref "Playback Controls.vi"() -> (w77:refnum<vi>)
  n173 = property class="VI"() -> ("Panel"=w79:refnum<vi>)  [unwired: 2 in, 2 out]
  n174 = property class="Pnl"(reference=w79) -> ("Panes[]"=w80:refnum<vi>[])  [unwired: 1 in, 2 out]
  n175 = Index Array(array=w80) -> (element=w78:refnum<vi>)  [unwired: 1 in]
  n176 = control-ref of="Test Tree"() -> (w81:refnum<vi>)
  n177 = while {
    tunnel: [w283] -> _
    tunnel: w81 -> [w282]
    tunnel: w77 -> [w281]
    tunnel: w76 -> [w280]
    tunnel: w75 -> [_]
    tunnel: w71 -> [w279]
    tunnel: w56 -> [w278]
    tunnel: w55 -> [w277]
    shift-right: [w276] -> _
    shift-left: _ -> [w275]
    tunnel: w52 -> [w274]
    i -> [w283]
    stop <- FALSE stop-if-true
    n178 = event shown="[0] Timeout" {
      selector: w280 -> [_ _ _ _ _ _ _ _ _ _ _ _ _ _ _ _ _]
      dyn-events: [_ _ _ _ _ _ _ _ _ _ _ _ w513 _ _ _ _] -> _
      timeout: u32 60 ("milliseconds to wait") -> [_ _ _ _ _ _ _ _ _ _ _ _ _ _ _ _ _]
      tunnel: w282 -> [w295 _ _ _ _ _ _ _ _ _ _ _ _ _ _ _ _]
      tunnel: "Test Tree" -> [_ _ _ _ _ _ _ w480 w488 w490 w494 w502 _ _ _ _ _]
      tunnel: w281 -> [_ _ _ _ _ _ _ _ _ _ _ _ w515 _ w533 _ _]
      tunnel: w279 -> [_ _ _ _ _ _ _ _ _ _ _ _ w511 _ _ _ _]
      tunnel: w278 -> [_ _ _ _ _ _ _ _ _ _ _ _ w509 _ _ _ _]
      tunnel: w277 -> [w290 _ _ _ w455 _ _ _ _ _ _ _ _ _ _ _ _]
      tunnel: [w289 w338 w440 w445 w453 w462 w472 w479 w486 w489 w493 w501 w508 w528 w530 w534 w547] -> w276
      tunnel: w275 -> [w289 w338 w440 w445 w453 _ _ w479 w486 w489 w493 w501 w508 w528 w530 w534 w547]
      tunnel: w274 -> [w287 _ _ _ _ _ _ _ _ _ _ _ _ _ _ _ _]
      event Timeout {
        n179 = event-data() -> ()  [unwired: 1 in, 1 out]
        n180 = local read "Mode"() -> (w292:T3)
        n181 = case shown="\"Test\"" "Dashboard Tab" {
          tunnel: w295 -> [_ _ w311 _ _]
          tunnel: "TestMode/Automatic/" ("Name Pattern") -> [_ _ w310 _ _]
          tunnel: T24 [{"Operation"=enum."Clear", "Color Box"=14013909}, {"Operation"=enum."Clear", "Color Box"=14013909}, {"Operation"=enum."Clear", "Color Box"=14013909}, {"Operation"=enum."Clear", "Color Box"=14013909}, {"Operation"=enum."Update", "Color Box"=14013909}, {"Operation"=enum."Update", "Color Box"=16777215}, {"Operation"=enum."Clear", "Color Box"=14013909}, {"Operation"=enum."Clear", "Color Box"=14013909}, {"Operation"=enum."Clear", "Color Box"=14013909}] -> [_ _ w303 _ w331]
          tunnel: w292 -> [_ _ w302 _ w330]
          tunnel: u32[] [15790320, 15790320, 15790320, 15790320, 16777215, 16777215, 15790320, 15790320, 15790320] -> [_ _ _ _ w336]
          tunnel: w290 -> [_ _ _ _ w324]
          tunnel: w287 -> [_ w297 _ _ _]
          frame "Custom", Default {
          }
          frame "Basic" {
            n182 = call <vilib>:"WPI_DashboardUpdateNames.vi"("Controls on Tab"=w297) -> ()  [unwired: 11 in]
          }
          frame "Test" {
            w309 = -2 ("Active Item:Row Number")
            n183 = Index Array(array=w303, index=w302) -> (element=w304:T26)
            n184 = Unbundle(w304) -> ("Operation"=w305:enum16{"Update", "Clear"}, "Color Box"=w306:u32)
            n185 = call <vilib>:"NT Read String.vi"("Name"="TestMode/TestName") -> ("String"=w300:string)  [unwired: 9 in, 1 out]
            n186 = call <vilib>:"NT Read and Format Entries as Tree.vi"("Operation"=w305, "Name Pattern"=w310, "Tree Refnum"=w311) -> ()  [unwired: 7 in, 2 out]
            n187 = case shown="\"\"" w300 {
              tunnel: "TestMode/TestProgress" ("Name") -> [w313 _]
              tunnel: "TestMode/TestProgressText" ("Name") -> [w312 _]
              frame Default {
                n188 = call <vilib>:"NT Read Number.vi"("Name"=w313) -> ("Numeric"=w314:dbl)  [unwired: 9 in, 1 out]
                n189 = call <vilib>:"NT Read String.vi"("Name"=w312) -> ("String"=w315:string)  [unwired: 9 in, 1 out]
                n190 = Bundle("Numeric"=w314, "String"=w315) -> (→"Progress":cluster{"Numeric":dbl, "String":string})  [unwired: 1 in]
              }
              frame "" {
                n191 = property on="Progress" class="Clust (strict)"("Visible"=FALSE) -> ()  [unwired: 2 in, 2 out]
                n192 = local write "Test Name"(u16 0) -> ()
              }
            }
            n193 = property on="Test Tree" class="Tree (strict)"("Active Item Row Number"=w309, "ActiveColNum"=w309, "CellBG"=w306, "Active Item Row Number"=-1 ("Active Item:Row Number"), "CellBG"=u32 5789784 ("Color Box")) -> ()  [unwired: 2 in, 2 out]
          }
          frame "Variables" {
            w321 = string[] ["CameraPublisher", "Usage", "DB"]  # Items to initially close
            n194 = First Call?() -> (First Call?: T/F=w322:bool)
            n195 = control-ref of="Tree"() -> (w323:refnum<vi>)
            n196 = Select(t=w321, s=w322, f=string[] []) -> (s? t:f=w319:string[])
            n197 = call <vilib>:"NT Read and Format Entries as Tree.vi"("Tags to  Close"=w319, "Tree Refnum"=w323) -> ()  [unwired: 8 in, 2 out]
          }
          frame "Commands" {
            w332 = u32 5789784 ("Color Box")
            w333 = T27 {"Row"=-1, "Column"=-2} ("Active Cell:Active Cell")
            w335 = T27 {"Row"=-2, "Column"=-2} ("Active Cell:Active Cell")
            n198 = Index Array(array=w336, index=w330) -> (element=w334:u32)
            n199 = Index Array(array=w331, index=w330) -> (element=w329:T26)
            n200 = Unbundle(w329) -> ("Operation"=w328:enum16{"Update", "Clear"})  [unwired: 1 out]
            n201 = local read "Command Selection"() -> (w327:i32)
            n202 = property on="Command Selection" class="MCListbox (strict)"("ActiveCell"=w335, "CellBG"=w334, "ActiveCell"=w333, "CellBG"=w332) -> ()  [unwired: 2 in, 2 out]
            n203 = call <vilib>:"WPI_DashboardUpdate RPC Info.vi"("Operation"=w328) -> ("update"=w326:bool, "commands"=w325:string[][])  [unwired: 9 in]
            n204 = property on="Command Selection" class="MCListbox (strict)"("ItemNames"=w325) -> ()  [unwired: 2 in, 2 out]
            n205 = property on="Command Params" class="Tbl (strict)"("Active Cell"=w335, "Cell BG Color"=w334, "Active Cell"=w333, "Cell BG Color"=w332) -> ()  [unwired: 2 in, 2 out]
            n206 = call <vilib>:"WPI_DashboardUpdate Command Params.vi"("Update"=w326, "NewVal"=w327, "Commands"=w325, "Param Tbl"=w324) -> ()  [unwired: 7 in, 1 out]
          }
        }
        n207 = call <vilib>:"Connextion Info.vi"() -> ("Connected"=→"NT Connection":bool)  [unwired: 10 in, 1 out]
      }
      event "Test Tree": Value Change {
        # "Show appropriate\ncontrols"
        n208 = event-data() -> ("CtlRef"=w341:refnum<vi>, "NewVal"=w339:string)  [unwired: 1 in]
        n209 = call <vilib>:"WPI_UtilitiesGetTreeIOName.vi"("NewVal"=w339, "TreeControl in"=w341) -> ("I/O Name"=w342:string)  [unwired: 9 in]
        n210 = case shown="\"Camera\"" w342 {
          selector: w342 -> [_ w349 _ w371 w380 _]
          tunnel: w339 -> [_ _ w368 w370 _ w387]
          tunnel: cluster{string[]}[] [{["640x480", "320x240", "160x120"]}, {["Auto", "Fixed indoor", "Fixed outdoor 1", "Fixed outdoor 2", "Fixed fluorescent 1", "Fixed fluorescent 2", "Hold current"]}, {["Auto", "Flicker-free 50 Hz", "Flicker-free 60 Hz", "Hold current"]}, {["None", "Prioritize frame rate", "Prioritize image quality"]}, {["Monochrome", "Color"]}] -> [_ _ _ _ _ w386]
          frame Default {
            w344 = FALSE ("Visible")
            w343 = FALSE ("Visible")
            n211 = property on="Motor" class="Clust (strict)"("Visible"=w343) -> ()  [unwired: 2 in, 2 out]
            n212 = property on="Test Ring" class="Ring (strict)"("Visible"=w343) -> ()  [unwired: 2 in, 2 out]
            n213 = property on="Rev/Fwd" class="Clust (strict)"("Visible"=w344) -> ()  [unwired: 2 in, 2 out]
            n214 = property on="On/Off" class="Bool (strict)"("Visible"=w344) -> ()  [unwired: 2 in, 2 out]
            n215 = property on="Test Slider" class="Slide (strict)"("Visible"=w344) -> ()  [unwired: 2 in, 2 out]
          }
          frame "Analog Out", "Motor", "PWM" {
            w350 = FALSE ("Visible")
            n216 = case shown="\"Analog Out\"" w349 {
              tunnel: [1.0 ("Value") -1.0 ("Value") 0.0 ("Value")] -> w348
              tunnel: [255.0 ("Value") 1.0 ("Value") 5.0 ("Value")] -> w347
              tunnel: [128.0 ("Value") 0.0 ("Value") 0.0 ("Value")] -> w346
              tunnel: [64.0 ("Value") 0.5 ("Value") 1.0 ("Value")] -> w345
              frame "PWM" {
              }
              frame "Motor", Default {
              }
              frame "Analog Out" {
              }
            }
            n217 = property on="Motor" class="Clust (strict)"("Visible"=TRUE) -> ()  [unwired: 2 in, 2 out]
            n218 = property on="Value" class="Slide (strict)"("Value"=w346, "Scale.Minimum"=w348, "Scale.Maximum"=w347, "Scale.Increment"=w345) -> ()  [unwired: 2 in, 2 out]
            n219 = property on="On/Off" class="Bool (strict)"("Visible"=w350) -> ()  [unwired: 2 in, 2 out]
            n220 = property on="Test Slider" class="Slide (strict)"("Visible"=w350) -> ()  [unwired: 2 in, 2 out]
            n221 = property on="Test Ring" class="Ring (strict)"("Visible"=w350) -> ()  [unwired: 2 in, 2 out]
            n222 = property on="Rev/Fwd" class="Clust (strict)"("Visible"=w350) -> ()  [unwired: 2 in, 2 out]
          }
          frame "Servo" {
            w366 = FALSE ("Visible")
            n223 = call <vilib>:"NT Read Number.vi"("Name"=w368) -> ("Numeric"=w367:dbl)  [unwired: 9 in, 1 out]
            n224 = property on="Test Slider" class="Slide (strict)"("Visible"=TRUE, "Scale.Maximum"=170.0 ("Scale.Range:Maximum")) -> ()  [unwired: 2 in, 2 out]
            n225 = local write "Test Slider"(w367) -> ()
            n226 = property on="Motor" class="Clust (strict)"("Visible"=w366) -> ()  [unwired: 2 in, 2 out]
            n227 = property on="Rev/Fwd" class="Clust (strict)"("Visible"=w366) -> ()  [unwired: 2 in, 2 out]
            n228 = property on="On/Off" class="Bool (strict)"("Visible"=w366) -> ()  [unwired: 2 in, 2 out]
            n229 = property on="Test Ring" class="Ring (strict)"("Visible"=w366) -> ()  [unwired: 2 in, 2 out]
          }
          frame "Relay", "Solenoid" {
            w369 = FALSE ("Visible")
            n230 = property on="Motor" class="Clust (strict)"("Visible"=w369) -> ()  [unwired: 2 in, 2 out]
            n231 = property on="Test Slider" class="Slide (strict)"("Visible"=w369) -> ()  [unwired: 2 in, 2 out]
            n232 = Search and Replace String(input string=w370, search string="/Value  **", replace string="/Direction") -> (result string=w376:string)  [unwired: 5 in, 3 out]
            n233 = property on="Test Ring" class="Ring (strict)"("Visible"=w369) -> ()  [unwired: 2 in, 2 out]
            n234 = call <vilib>:"NT Read String.vi"("Name"=w376) -> ("String"=w374:string)  [unwired: 9 in, 1 out]
            n235 = Equal?(x="Both directions", y=w374) -> (x = y?=w372:bool)
            n236 = Not(x=w372) -> (.not. x?=w373:bool)
            n237 = property on="Rev/Fwd" class="Clust (strict)"("Visible"=w372) -> ()  [unwired: 2 in, 2 out]
            n238 = property on="On/Off" class="Bool (strict)"("Visible"=w373, "Caption.Text"=w371) -> ()  [unwired: 2 in, 2 out]
          }
          frame "Compressor", "Digital Out" {
            w379 = FALSE ("Visible")
            # "Get direction and finish"
            n239 = property on="Motor" class="Clust (strict)"("Visible"=w379) -> ()  [unwired: 2 in, 2 out]
            n240 = property on="Test Slider" class="Slide (strict)"("Visible"=w379) -> ()  [unwired: 2 in, 2 out]
            n241 = property on="Test Ring" class="Ring (strict)"("Visible"=w379) -> ()  [unwired: 2 in, 2 out]
            n242 = property on="On/Off" class="Bool (strict)"("Visible"=TRUE, "Caption.Text"=w380) -> ()  [unwired: 2 in, 2 out]
            n243 = property on="Rev/Fwd" class="Clust (strict)"("Visible"=FALSE) -> ()  [unwired: 2 in, 2 out]
          }
          frame "Camera" {
            n244 = call <vilib>:"Get Last Path Segment.vi"("String in"=w387) -> ("String out"=w388:string)  [unwired: 10 in]
            n245 = property on="On/Off" class="Bool (strict)"("Visible"=FALSE) -> ()  [unwired: 2 in, 2 out]
            n246 = property on="Motor" class="Clust (strict)"("Visible"=FALSE) -> ()  [unwired: 2 in, 2 out]
            n247 = property on="Rev/Fwd" class="Clust (strict)"("Visible"=FALSE) -> ()  [unwired: 2 in, 2 out]
            n248 = case shown="\"White Balance  **\"" w388 {
              tunnel: w387 -> [w394 w403 w412 w421 w430 _ w436]
              tunnel: w386 -> [w392 w400 w409 w418 w427 _ _]
              frame "Size  **" {
                n249 = Index Array(array=w392) -> (element=w391:cluster{string[]})  [unwired: 1 in]
                n250 = call <vilib>:"NT Read String.vi"("Name"=w394) -> ("String"=w393:string)  [unwired: 9 in, 1 out]
                n251 = Unbundle(w391) -> (w389:string[])
                n252 = Match First String(2:w389, 3:w393) -> (0:w390:i32)  [unwired: 1 out]
                n253 = property on="Test Ring" class="Ring (strict)"("Value"=w390, "Strings []"=w389) -> ()  [unwired: 2 in, 2 out]
                n254 = property on="Test Ring" class="Ring (strict)"("Visible"=TRUE) -> ()  [unwired: 2 in, 2 out]
                n255 = property on="Test Slider" class="Slide (strict)"("Visible"=FALSE) -> ()  [unwired: 2 in, 2 out]
              }
              frame "White Balance  **" {
                n256 = Index Array(array=w400, index=1) -> (element=w401:cluster{string[]})
                n257 = call <vilib>:"NT Read String.vi"("Name"=w403) -> ("String"=w402:string)  [unwired: 9 in, 1 out]
                n258 = Unbundle(w401) -> (w398:string[])
                n259 = Match First String(2:w398, 3:w402) -> (0:w397:i32)  [unwired: 1 out]
                n260 = property on="Test Ring" class="Ring (strict)"("Value"=w397, "Strings []"=w398) -> ()  [unwired: 2 in, 2 out]
                n261 = property on="Test Ring" class="Ring (strict)"("Visible"=TRUE) -> ()  [unwired: 2 in, 2 out]
                n262 = property on="Test Slider" class="Slide (strict)"("Visible"=FALSE) -> ()  [unwired: 2 in, 2 out]
              }
              frame "Exposure  **" {
                n263 = Index Array(array=w409, index=2) -> (element=w410:cluster{string[]})
                n264 = call <vilib>:"NT Read String.vi"("Name"=w412) -> ("String"=w411:string)  [unwired: 9 in, 1 out]
                n265 = Unbundle(w410) -> (w406:string[])
                n266 = Match First String(2:w406, 3:w411) -> (0:w407:i32)  [unwired: 1 out]
                n267 = property on="Test Ring" class="Ring (strict)"("Value"=w407, "Strings []"=w406) -> ()  [unwired: 2 in, 2 out]
                n268 = property on="Test Ring" class="Ring (strict)"("Visible"=TRUE) -> ()  [unwired: 2 in, 2 out]
                n269 = property on="Test Slider" class="Slide (strict)"("Visible"=FALSE) -> ()  [unwired: 2 in, 2 out]
              }
              frame "Exposure Priority  **" {
                n270 = Index Array(array=w418, index=3) -> (element=w419:cluster{string[]})
                n271 = call <vilib>:"NT Read String.vi"("Name"=w421) -> ("String"=w420:string)  [unwired: 9 in, 1 out]
                n272 = Unbundle(w419) -> (w415:string[])
                n273 = Match First String(2:w415, 3:w420) -> (0:w416:i32)  [unwired: 1 out]
                n274 = property on="Test Ring" class="Ring (strict)"("Value"=w416, "Strings []"=w415) -> ()  [unwired: 2 in, 2 out]
                n275 = property on="Test Ring" class="Ring (strict)"("Visible"=TRUE) -> ()  [unwired: 2 in, 2 out]
                n276 = property on="Test Slider" class="Slide (strict)"("Visible"=FALSE) -> ()  [unwired: 2 in, 2 out]
              }
              frame "Color Enable  **" {
                n277 = Index Array(array=w427, index=4) -> (element=w428:cluster{string[]})
                n278 = call <vilib>:"NT Read String.vi"("Name"=w430) -> ("String"=w429:string)  [unwired: 9 in, 1 out]
                n279 = Unbundle(w428) -> (w424:string[])
                n280 = Match First String(2:w424, 3:w429) -> (0:w425:i32)  [unwired: 1 out]
                n281 = property on="Test Ring" class="Ring (strict)"("Value"=w425, "Strings []"=w424) -> ()  [unwired: 2 in, 2 out]
                n282 = property on="Test Ring" class="Ring (strict)"("Visible"=TRUE) -> ()  [unwired: 2 in, 2 out]
                n283 = property on="Test Slider" class="Slide (strict)"("Visible"=FALSE) -> ()  [unwired: 2 in, 2 out]
              }
              frame Default {
                n284 = property on="Test Ring" class="Ring (strict)"("Visible"=FALSE) -> ()  [unwired: 2 in, 2 out]
                n285 = property on="Test Slider" class="Slide (strict)"("Visible"=FALSE) -> ()  [unwired: 2 in, 2 out]
              }
              frame "Brightness  **", "Color Level  **", "Compression  **", "FPS  **", "Sharpness  **" {
                n286 = call <vilib>:"NT Read Number.vi"("Name"=w436) -> ("Numeric"=w435:dbl)  [unwired: 9 in, 1 out]
                n287 = local write "Test Slider"(w435) -> ()
                n288 = property on="Test Slider" class="Slide (strict)"("Visible"=TRUE, "Scale.Maximum"=100.0 ("Scale.Range:Maximum")) -> ()  [unwired: 2 in, 2 out]
                n289 = property on="Test Ring" class="Ring (strict)"("Visible"=FALSE) -> ()  [unwired: 2 in, 2 out]
              }
            }
          }
        }
        n290 = property on="Progress" class="Clust (strict)"("Visible"=FALSE) -> ()  [unwired: 2 in, 2 out]
      }
      event "Test Name": Mouse Enter {
        # "Populate the ring with the list of tests"
        n291 = event-data() -> ()  [unwired: 1 in, 1 out]
        n292 = call <vilib>:"NT Read String Array.vi"("Name"="TestMode/TestList") -> ("String Array"=w444:string[])  [unwired: 9 in, 1 out]
        n293 = Build Array (concatenate)("Select the test to run...", w444) -> (w443:string[])
        n294 = property on="Test Name" class="Ring (strict)"("Strings []"=w443) -> ()  [unwired: 2 in, 2 out]
      }
      event "Test Name": Value Change {
        w446 = FALSE ("Visible")
        # "Tell the robot the test name to run"
        n295 = event-data() -> ("NewVal"=w450:u16)  [unwired: 1 in]
        n296 = property on="Test Name" class="Ring (strict)"() -> ("Strings []"=w451:string[])  [unwired: 2 in, 2 out]
        n297 = local write "Progress"(T5 {"Test Progress"=0, "Test Progress Text"=""} ("Progress")) -> ()
        n298 = Index Array(array=w451, index=w450) -> (element=w449:string)
        n299 = call <vilib>:"NT Write String.vi"("String"=w449, "Name"="TestMode/TestName") -> ()  [unwired: 9 in, 1 out]
        n300 = property on="Progress" class="Clust (strict)"("Visible"=TRUE) -> ()  [unwired: 2 in, 2 out]
        n301 = property on="Motor" class="Clust (strict)"("Visible"=w446) -> ()  [unwired: 2 in, 2 out]
        n302 = property on="Test Slider" class="Slide (strict)"("Visible"=w446) -> ()  [unwired: 2 in, 2 out]
        n303 = property on="On/Off" class="Bool (strict)"("Visible"=w446) -> ()  [unwired: 2 in, 2 out]
        n304 = property on="Rev/Fwd" class="Clust (strict)"("Visible"=w446) -> ()  [unwired: 2 in, 2 out]
        n305 = property on="Test Ring" class="Ring (strict)"("Visible"=w446) -> ()  [unwired: 2 in, 2 out]
      }
      event "Command Selection": Value Change {
        # "Get the params and show in table"
        n306 = event-data() -> ("NewVal"=w456:i32)  [unwired: 1 in]
        n307 = property on="Command Selection" class="MCListbox (strict)"() -> ("ItemNames"=w454:string[][])  [unwired: 2 in, 2 out]
        n308 = call <vilib>:"WPI_DashboardUpdate Command Params.vi"("NewVal"=w456, "Commands"=w454, "Param Tbl"=w455) -> ()  [unwired: 8 in, 1 out]
      }
      event "Execute Command": Value Change {
        # "Started one, Unique ID holds\nresponse"
        n309 = event-data() -> ()  [unwired: 1 in, 1 out]
        n310 = property on="Command Selection" class="MCListbox (strict)"() -> ("ItemNames"=w467:string[][])  [unwired: 2 in, 2 out]
        n311 = Index Array(array=w467, index (row)="Command Selection", index (col)=0) -> (element=w465:string)
        n312 = call <vilib>:"Invoke Commands.vi"("Command Params"="Command Params", "Function Name"=w465) -> ("Params"=w461:u8, "Started"=w460:bool)  [unwired: 7 in, 1 out]
        n313 = Array Subset(array="Command Params", length (row)=w461) -> (w462:string[][])  [unwired: 3 in]
        n314 = Select(t="Executing" ("Cmd Status"), s=w460, f="" ("Cmd Status")) -> (s? t:f=→"Cmd Status":string)
      }
      event "Command Selection": Double Click {
        n315 = event-data() -> ("Row"=w475:i32)  [unwired: 1 in]
        n316 = property on="Command Selection" class="MCListbox (strict)"() -> ("ItemNames"=w478:string[][])  [unwired: 2 in, 2 out]
        n317 = local read "Command Params"() -> (w474:string[][])
        n318 = Index Array(array=w478, index (row)=w475, index (col)=0) -> (element=w476:string)
        n319 = call <vilib>:"Invoke Commands.vi"("Command Params"=w474, "Function Name"=w476) -> ("Params"=w473:u8, "Started"=w468:bool)  [unwired: 7 in, 1 out]
        n320 = Array Subset(array=w474, length (row)=w473) -> (w472:string[][])  [unwired: 3 in]
        n321 = Select(t="Executing" ("Cmd Status"), s=w468, f="" ("Cmd Status")) -> (s? t:f=w469:string)
        n322 = local write "Cmd Status"(w469) -> ()
      }
      event "Motor.Enable": Value Change {
        # "When the test mode otor enable helper is set, update that\ntree row item's value"
        n323 = event-data() -> ("NewVal"=w484:bool)  [unwired: 1 in]
        n324 = Unbundle("Motor") -> ("Value"=w483:dbl)  [unwired: 1 out]
        n325 = Select(t=w483, s=w484, f=0.0) -> (s? t:f=w481:dbl)
        n326 = call <vilib>:"NT Write Number.vi"("Numeric"=w481, "Name"=w480) -> ()  [unwired: 9 in, 1 out]
      }
      event "Test Slider": Value Change {
        # "When the test mode slider helper is set, update that\ntree row item's value"
        n327 = event-data() -> ("NewVal"=w487:dbl)  [unwired: 1 in]
        n328 = call <vilib>:"NT Write Number.vi"("Numeric"=w487, "Name"=w488) -> ()  [unwired: 9 in, 1 out]
      }
      event "On/Off": Value Change {
        # "When the test mode on/off helper value is set, update that\ntree row item's value"
        n329 = event-data() -> ("NewVal"=w492:bool)  [unwired: 1 in]
        n330 = Boolean To (0,1)(Boolean=w492) -> (0, 1=w491:i16)
        n331 = call <vilib>:"NT Write Number.vi"("Numeric"=w491, "Name"=w490) -> ()  [unwired: 9 in, 1 out]
      }
      event "Rev/Fwd": Value Change {
        # "When the test mode helper value for relays is set, update that\ntree row item's value"
        n332 = event-data() -> ("NewVal.Forward"=w500:bool, "NewVal.Reverse"=w499:bool)  [unwired: 1 in]
        n333 = Boolean To (0,1)(Boolean=w500) -> (0, 1=w496:i16)
        n334 = Boolean To (0,1)(Boolean=w499) -> (0, 1=w498:i16)
        n335 = Negate(x=w498) -> (-x=w497:i16)
        n336 = Add(x=w496, y=w497) -> (x+y=w495:i16)
        n337 = call <vilib>:"NT Write Number.vi"("Numeric"=w495, "Name"=w494) -> ()  [unwired: 9 in, 1 out]
      }
      event "Test Ring": Value Change {
        # "When a test mode helper value is selected from the ring,\nset the tree item's variable to the string value"
        n338 = event-data() -> ("NewVal"=w504:u16)  [unwired: 1 in]
        n339 = property on="Test Ring" class="Ring (strict)"() -> ("Strings []"=w505:string[])  [unwired: 2 in, 2 out]
        n340 = Index Array(array=w505, index=w504) -> (element=w503:string)
        n341 = call <vilib>:"NT Write String.vi"("String"=w503, "Name"=w502) -> ()  [unwired: 9 in, 1 out]
      }
      event "Rec Mode": Value Change {
        # "Update globals for recording mode and path to read log from.\nClear when logging and let NetworkTables set path for vision to\nuse."
        n342 = event-data() -> ("NewVal"=w516:enum32{"Stop", "Record", "Playback"})  [unwired: 1 in]
        n343 = global write "WPI_DashboardLogging Global.vi" "Logging Filename"(path "") -> ()
        n344 = global write "WPI_DashboardLogging Global.vi" "Recording"(w516) -> ()
        n345 = case shown="\"Playback\"" w516 {
          tunnel: w515 -> [_ w518 w527]
          tunnel: [_ _ w526] -> w513
          tunnel: [_ _ w525] -> _
          tunnel: w511 -> [_ _ w523]
          tunnel: cluster{i32, i32} {-250, 170} -> [_ _ w522]
          tunnel: [_ _ T25 {"Image Size"=TRUE, "Image Type"=TRUE, "Pixel Value"=TRUE, "ROI Information"=TRUE, "Zoom Factor"=FALSE} ("Image Information Shown:All Elements")] -> w506
          tunnel: [_ _ TRUE ("Zoom Factor")] -> w507
          tunnel: w509 -> [_ _ w519]
          frame Default {
          }
          frame "Stop", "Record" {
            # "Place Window too"
            n346 = invoke class="VI" method="FP.Close"(reference=w518) -> (reference out=w517:refnum<vi>)  [unwired: 2 in, 2 out]
            n347 = invoke class="VI" method="Abort VI"(reference=w517) -> ()  [unwired: 2 in, 3 out]
          }
          frame "Playback" {
            n348 = call "Open Playback Panel.vi"("Offset"=w522, "DB VI Ref"=w523, "Playback in"=w527) -> ("Playback out"=w524:refnum<vi>)  [unwired: 8 in]
            n349 = register-events(w524, w519) -> (reference out=w526:refnum<event-registration>, error out=w525:errorcluster)  [unwired: 2 in]
          }
        }
        n350 = property on="Camera Image" class="ImageControl"("Image Information Shown"=w506, "Image Information Visible"=w507) -> ()  [unwired: 2 in, 2 out]
        n351 = call <vilib>:"WPI_DashboardNT Log FieldName Cache.vi"("Operation"=enum16{"Lookup/Add", "Index", "Clear"}."Clear") -> ()  [unwired: 8 in, 3 out]
      }
      event Panel Close {
        w529 = enum32{"Stop", "Record", "Playback"}."Stop" ("Rec Mode")
        # "Playback window has been closed, abort"
        n352 = event-data() -> ()  [unwired: 1 in, 4 out]
        n353 = local write "Rec Mode"(w529) -> ()
        n354 = global write "WPI_DashboardLogging Global.vi" "Recording"(w529) -> ()
      }
      event Panel Close {
        # "Abort playback window and ourself"
        n355 = event-data() -> ()  [unwired: 1 in, 4 out]
        n356 = invoke class="VI" method="FP.Close"(reference=w533) -> (reference out=w532:refnum<vi>)  [unwired: 2 in, 2 out]
        n357 = invoke class="VI" method="Abort VI"(reference=w532) -> (error out=w531:errorcluster)  [unwired: 2 in, 2 out]
        n358 = invoke class="VI" method="Abort VI"(error in=w531) -> ()  [unwired: 2 in, 3 out]
      }
      event User Event {
        n359 = event-data() -> ("IDs"=w540:cluster{"RPC field ID":u16, "Unique ID":u16}, "String"=w539:string)  [unwired: 1 in]
        n360 = Bundle("IDs"=w540, "String"=w539) -> (w538:T10)  [unwired: 1 in]
        n361 = call <vilib>:"Retrieve RPC Response.vi"("RPC Response"=w538) -> ("Output"=w536:string[][])  [unwired: 10 in]
        n362 = Build Array (concatenate)(w534, w536) -> (w535:string[][])
        n363 = local write "Command Params"(w535) -> ()
        n364 = local write "Cmd Status"("" ("Cmd Status")) -> ()
      }
      event "Tree": Double Click {
        n365 = event-data() -> ("PlatMods"=w546:T28, "Tag"=w543:string)  [unwired: 1 in]
        n366 = Unbundle(w546) -> ("Shift"=w545:bool)  [unwired: 4 out]
        n367 = String Subset(string=w543, length (rest)=1 ("length (rest)")) -> (substring=w542:string)  [unwired: 1 in]
        n368 = Not(x=w545) -> (.not. x?=w544:bool)
        n369 = case shown="\"/\"" w542 {
          tunnel: w543 -> [_ w549]
          tunnel: w544 -> [_ w548]
          frame Default {
          }
          frame "/" {
            n370 = call <vilib>:"NT Update Persistence.vi"("Persistence"=w548, "Name"=w549) -> ()  [unwired: 9 in, 1 out]
          }
        }
      }
    }
  }
  n371 = while {
    tunnel: w78 -> [w551]
    i -> [w554]
    stop <- FALSE stop-if-true
    n372 = Wait (ms)(milliseconds to wait=u32 100) -> ()  [unwired: 1 out]
    n373 = case shown="\"Playback\"" "Rec Mode" {
      tunnel: w554 -> [_ _ w569]
      tunnel: [u32 2829099 ("Base Color") u32 11141120 ("Target Color") w558] -> w550
      frame "Stop", Default {
        # "Reset the color, extra updates don't cost much"
      }
      frame "Record" {
      }
      frame "Playback" {
        # "Playback"
        n374 = Quotient & Remainder(x=w569, y=u32 50 ("milliseconds to wait")) -> (x-y*floor(x/y)=w565:u32)  [unwired: 1 out]
        n375 = Divide(x=w565, y=u32 50 ("milliseconds to wait")) -> (x/y=w562:dbl)
        n376 = Multiply(x=6.283185307179586, y=w562) -> (x*y=w567:dbl)
        n377 = Sine(x=w567) -> (sin(x)=w566:dbl)
        n378 = Absolute Value(x=w566) -> (abs(x)=w559:dbl)
        n379 = call "Interpolate RGB Color.vi"("Proportion"=w559, "Target Color"=u32 30976, "Base Color"=u32 2829099) -> ("Result Color"=w558:u32)  [unwired: 8 in]
      }
    }
    n380 = property class="Pane"(reference=w551, "PaneColor"=w550) -> ()  [unwired: 1 in, 2 out]
  }
  n381 = local write "Dashboard Tab"(T2."Variables" ("Dashboard Tab")) -> ()
  n382 = property on="On/Off" class="Bool (strict)"("Visible"=w64) -> ()  [unwired: 2 in, 2 out]
  n383 = property on="Motor" class="Clust (strict)"("Visible"=w64) -> ()  [unwired: 2 in, 2 out]
  n384 = property on="Progress" class="Clust (strict)"("Visible"=w64) -> ()  [unwired: 2 in, 2 out]
  n385 = property on="Test Ring" class="Ring (strict)"("Visible"=w64) -> ()  [unwired: 2 in, 2 out]
  n386 = property on="Rev/Fwd" class="Clust (strict)"("Visible"=w64) -> ()  [unwired: 2 in, 2 out]
  n387 = while {
    tunnel: u16 1741 ("timeout ms (25000)") -> [w571]
    stop <- FALSE stop-if-true
    n388 = TCP Create Listener(10:w571) -> (0:w570:errorcluster, 3:w572:refnum<k5>)  [unwired: 4 in, 1 out]
    n389 = case shown="No Error" w570 {
      selector: w570 -> [w574 _]
      tunnel: w572 -> [w575 _]
      frame No Error {
        n390 = while {
          tunnel: w575 -> [w578]
          tunnel: w574 -> [w577]
          stop <- FALSE stop-if-true
          n391 = TCP Wait On Listener(8:w577, 11:w578) -> (0:w579:errorcluster, 4:w580:refnum<k5>)  [unwired: 2 in, 3 out]
          n392 = local write "TCP"(w580) -> ()
          n393 = case shown="No Error" w579 {
            frame No Error {
            }
            frame Error {
              n394 = Wait (ms)(milliseconds to wait=u32 1000) -> ()  [unwired: 1 out]
            }
          }
        }
      }
      frame Error {
        n395 = Wait (ms)(milliseconds to wait=u32 1000) -> ()  [unwired: 1 out]
      }
    }
  }
  n396 = local write "Command Selection"(u16 0 ("milliseconds to wait")) -> ()
  n397 = local write "Command Params"(string[][] [] ("Command Params")) -> ()
  n398 = global write "WPI_DashboardLogging Global.vi" "Recording"(w72) -> ()
  n399 = local write "Rec Mode"(w72) -> ()
  n400 = call <vilib>:"NT Write String.vi"("Name"="Auto Selector") -> ()  [unwired: 10 in, 1 out]
